vi "WebServiceLoop.vi"(8 "Error In":errorcluster, 11 "Message Queues":T1) -> (0 "Error Out":errorcluster)   [LabVIEW 2017, in "Server.lvlib" / "WebServiceCommunication.lvlib"]
doc: "This Loop sets, reads and calls the WebServiceFGV.vi which is responsible for communicating with the Webservice Methods.\nThis Loop has a timeout on the queue read function and will call the \"CheckClients\"-mode of the FGV frequently to validate which clients are still sending their heartbeat.\nIt is waiting for Messages in the WebServ-Queue and forwards messages (such as current clients connected to the MHL)."
uses:
  WebServiceCommunication.lvlib
  Message Queue/CommReferences.ctl
  Message Queue/MessageCluster.ctl
  WebServiceLoopData.ctl
  TypeDefs/ClientConfiguration.ctl
  WebServiceFGVcommands.ctl
  TypeDefs/SR List.ctl
  TypeDefs/SR Data.ctl
  TypeDefs/ServerINI.ctl
  Oracle/OracleData.ctl
  <vilib>/Utility/error.llb/Error Cluster From Error Code.vi
  Message Queue/EnqueueMessage(Single).vi
  <vilib>/ErrorRing/Error Ring.xnode
  Message Queue/Message Queue.lvlib
  Server.lvlib
  ErrorLogger/ErrorLogger.lvlib
  Oracle/Oracle.lvlib
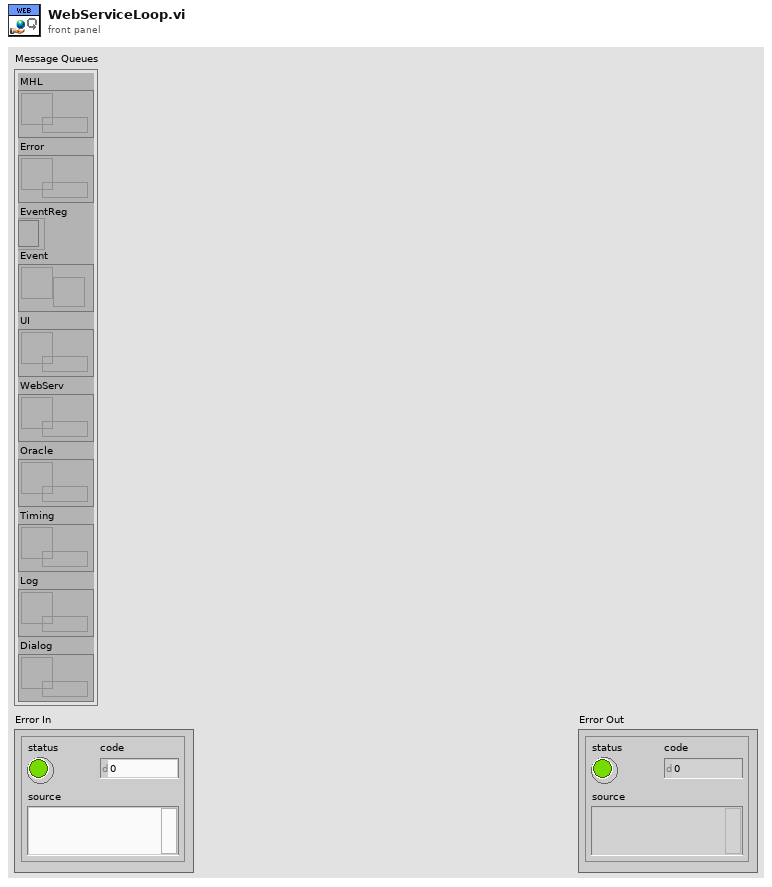
[diagram p1: front panel]
types:
  T1 = typedef "Server.lvlib/Message Queue.lvlib/CommReferences.ctl" = cluster{"MHL":refnum<queue>, "Error":refnum<queue>, "EventReg":refnum<event-registration>, "Event":refnum<user-event>, "UI":refnum<queue>, "WebServ":refnum<queue>, "Oracle":refnum<queue>, "Timing":refnum<queue>, "Log":refnum<queue>, "Dialog":refnum<queue>}
  T2 = typedef "Server.lvlib/WebServiceCommunication.lvlib/WebServiceLoopData.ctl" = cluster{"ClientTimeout":u32, "ClientConfig":T3}
  T3 = typedef "Server.lvlib/ClientConfiguration.ctl" = cluster{"ColorCodes":u32[]}
  T4 = typedef "Server.lvlib/WebServiceCommunication.lvlib/WebServiceFGVcommands.ctl" = enum16{"Init", "Reset", "Heartbeat", "GetSRs", "SetSRs", "CheckClients", "GetClients", "SetClientConfig", "GetClientConfig"}
  T5 = typedef "Server.lvlib/ServerINI.ctl" = cluster{"ClientTimeout (s)":u32, "LogPath":path, "ErrorsToIgnore":i32[], "OracleData":T6, "ClientConfig":T3}
  T6 = typedef "Server.lvlib/Oracle.lvlib/OracleData.ctl" = cluster{"DBname":string, "User":string, "Password":string}
  T7 = typedef "Server.lvlib/SR List.ctl" = T8[]
  T8 = typedef "Server.lvlib/SR Data.ctl" = cluster{"SR#":dbl, "Group":string, "Owner":string, "Problem Summary":string, "Last Updated":timestamp, "Customer First Name":string, "Customer Last Name":string, "Company":string, "Created On":timestamp, "SR Type":string, "Status":string, "Service Level":string, "Channel":string, "Days Open":dbl}
  T9 = typedef "Server.lvlib/ClientList.ctl" = T10[]
  T10 = typedef "Server.lvlib/ClientData.ctl" = cluster{"ClientID":string, "LastHeartbeat":timestamp}
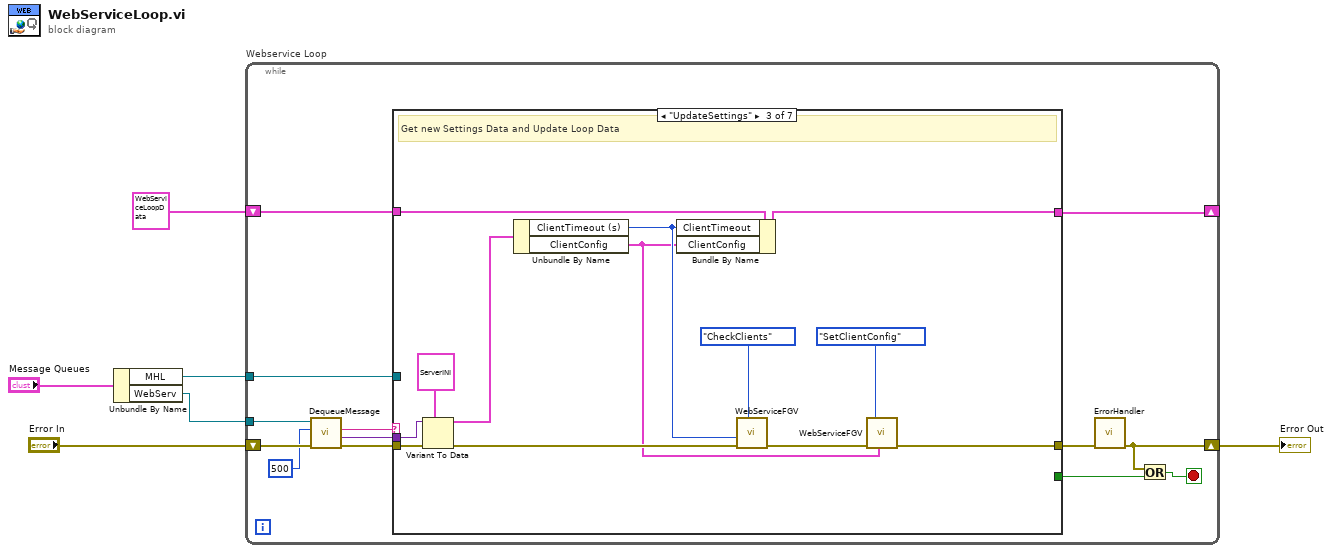
[diagram p0: block diagram]
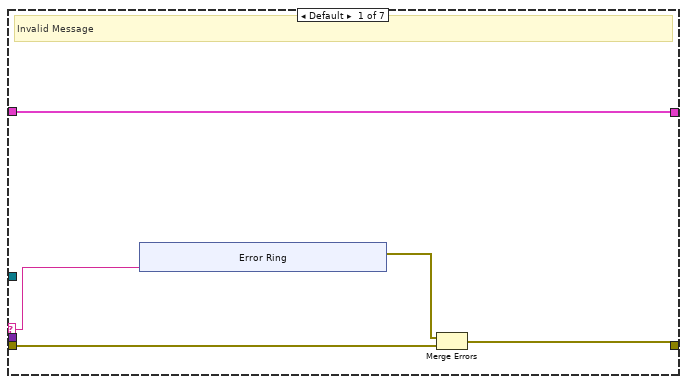
[diagram p2: hidden frame]
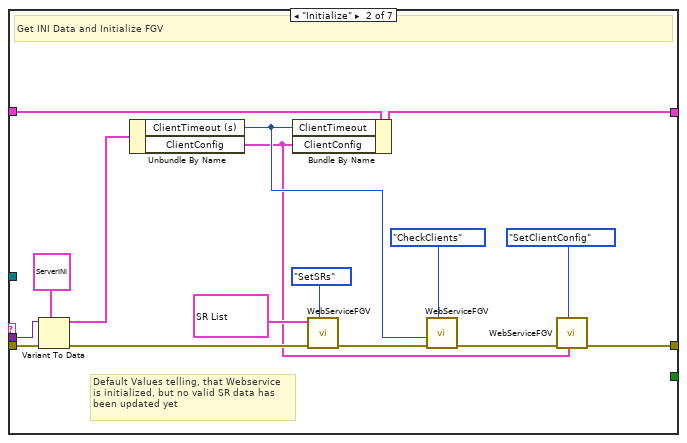
[diagram p3: hidden frame]
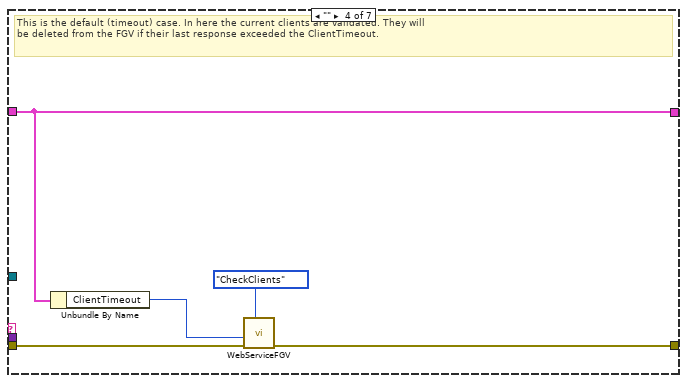
[diagram p4: hidden frame]
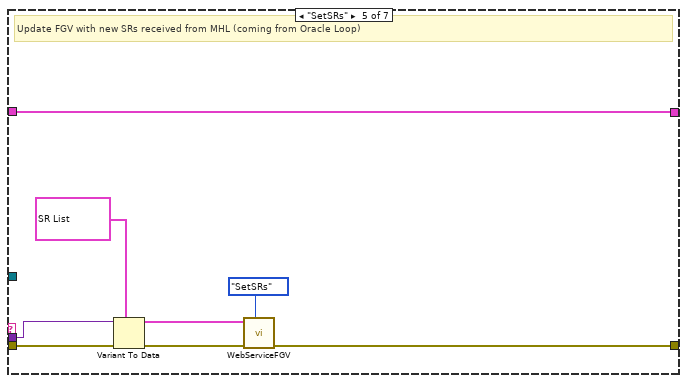
[diagram p5: hidden frame]
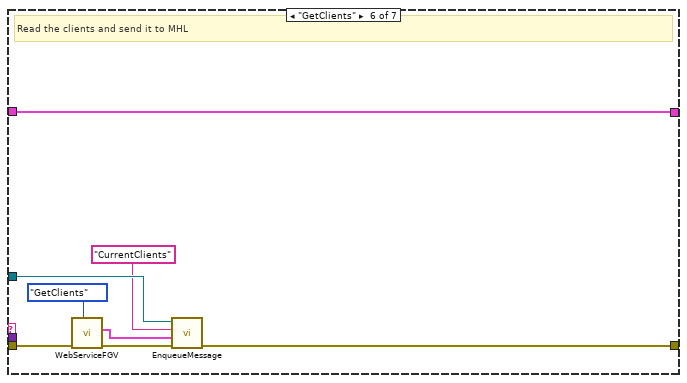
[diagram p6: hidden frame]
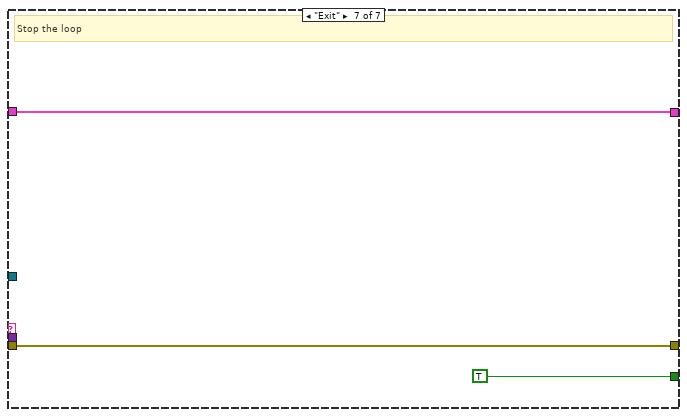
[diagram p7: hidden frame]
diagram:
  n1 = Unbundle By Name("Message Queues") -> ("MHL"=w2:refnum<queue>, "WebServ"=w3:refnum<queue>)
  n2 = while "Webservice Loop" {
    shift-right: [w7] -> w5
    shift-left: "Error In" -> [w19]
    tunnel: w3 -> [w16]
    tunnel: w2 -> [w11]
    shift-right: [w9] -> _
    shift-left: T2 {"ClientTimeout"=0, "ClientConfig"={"ColorCodes"=[16711680, 6618880, 16774745, 9567230]}} ("WebServiceLoopData") -> [w10]
    stop <- w8 stop-if-true
    n3 = call "DequeueMessage.vi"("error in (no error)"=w19, "timeout ms (-1)"=500, "Message Queue"=w16) -> ("error out"=w17:errorcluster, "Message Data"=w14:variant, "Message"=w15:string)  [unwired: 4 in, 2 out]
    n4 = case shown="\"UpdateSettings\"" w15 {
      selector: w15 -> [w21 _ _ _ _ _ _]
      tunnel: [w23 w34 w50 w61 w72 w78 w84] -> w18
      tunnel: w17 -> [w24 w47 w60 w65 w73 w81 w84]
      tunnel: w14 -> [_ w39 w57 _ w70 _ _]
      tunnel: [_ _ _ _ _ _ TRUE] -> w13
      tunnel: w11 -> [_ _ _ _ _ w77 _]
      tunnel: [w20 w38 w56 w63 w66 w74 w82] -> w9
      tunnel: w10 -> [w20 w42 w59 w63 w66 w74 w82]
      frame Default {
        # "Invalid Message"
        n5 = xnode "Error Ring"("parameter 0"=w21) -> ("error out"=w22:errorcluster)
        n6 = Merge Errors(w22, w24) -> (w23:errorcluster)
      }
      frame "Initialize" {
        # "Default Values telling, that Webservice\nis initialized, but no valid SR data has\nbeen updated yet"
        # "Get INI Data and Initialize FGV"
        n7 = Variant To Data(error in=w47, type=T5 {"ClientTimeout (s)"=30, "LogPath"=path "C:/Users/jgoebel/Documents/GitHub/AEDashboard/ServerLib/Data/ServerLog.tdms", "ErrorsToIgnore"=[], "OracleData"={"DBname"="", "User"="", "Password"=""}, "ClientConfig"={"ColorCodes"=[16711680, 6618880, 16774745, 9567230]}} ("ServerINI"), Variant=w39) -> (data=w37:T5, error out=w41:errorcluster)
        n8 = Unbundle By Name(w37) -> ("ClientTimeout (s)"=w36:u32, "ClientConfig"=w33:T3)
        n9 = Bundle By Name(cluster=w42, "ClientTimeout"=w36, "ClientConfig"=w33) -> (w38:T2)
        n10 = call "WebServiceFGV.vi"("CMD"=WebServiceFGVcommands."SetSRs", "error in (no error)"=w41, "SRListIn"=T7 [{"SR#"=1234.0, "Group"="THIS IS A DUMMY SR!", "Owner"="WEBSERVER IS INITIALIZED!", "Problem Summary"="BUT NO VALID SR DATA IS SET YET!", "Last Updated"=timestamp(0 s since 1904-01-01), "Customer First Name"="", "Customer Last Name"="", "Company"="", "Created On"=timestamp(0 s since 1904-01-01), "SR Type"="", "Status"="", "Service Level"="", "Channel"="", "Days Open"=0.0}]) -> ("error out"=w44:errorcluster)  [unwired: 5 in, 3 out]
        n11 = call "WebServiceFGV.vi"("CMD"=WebServiceFGVcommands."CheckClients", "error in (no error)"=w44, "ClientTimeout(s)(30)"=w36) -> ("error out"=w35:errorcluster)  [unwired: 5 in, 3 out]
        n12 = call "WebServiceFGV.vi"("ClientConfig"=w33, "CMD"=WebServiceFGVcommands."SetClientConfig", "error in (no error)"=w35) -> ("error out"=w34:errorcluster)  [unwired: 5 in, 3 out]
      }
      frame "UpdateSettings" {
        # "Get new Settings Data and Update Loop Data"
        n13 = Variant To Data(error in=w60, type=T5 {"ClientTimeout (s)"=30, "LogPath"=path "C:/Users/jgoebel/Documents/GitHub/AEDashboard/ServerLib/Data/ServerLog.tdms", "ErrorsToIgnore"=[], "OracleData"={"DBname"="", "User"="", "Password"=""}, "ClientConfig"={"ColorCodes"=[16711680, 6618880, 16774745, 9567230]}} ("ServerINI"), Variant=w57) -> (data=w55:T5, error out=w51:errorcluster)
        n14 = Unbundle By Name(w55) -> ("ClientTimeout (s)"=w49:u32, "ClientConfig"=w48:T3)
        n15 = Bundle By Name(cluster=w59, "ClientTimeout"=w49, "ClientConfig"=w48) -> (w56:T2)
        n16 = call "WebServiceFGV.vi"("CMD"=WebServiceFGVcommands."CheckClients", "error in (no error)"=w51, "ClientTimeout(s)(30)"=w49) -> ("error out"=w54:errorcluster)  [unwired: 5 in, 3 out]
        n17 = call "WebServiceFGV.vi"("ClientConfig"=w48, "CMD"=WebServiceFGVcommands."SetClientConfig", "error in (no error)"=w54) -> ("error out"=w50:errorcluster)  [unwired: 5 in, 3 out]
      }
      frame "" {
        # "This is the default (timeout) case. In here the current clients are validated. They will\nbe deleted from the FGV if their last response exceeded the ClientTimeout."
        n18 = Unbundle By Name(w63) -> ("ClientTimeout"=w62:u32)
        n19 = call "WebServiceFGV.vi"("CMD"=WebServiceFGVcommands."CheckClients", "error in (no error)"=w65, "ClientTimeout(s)(30)"=w62) -> ("error out"=w61:errorcluster)  [unwired: 5 in, 3 out]
      }
      frame "SetSRs" {
        # "Update FGV with new SRs received from MHL (coming from Oracle Loop)"
        n20 = Variant To Data(error in=w73, type=T7 [{"SR#"=0.0, "Group"="", "Owner"="", "Problem Summary"="", "Last Updated"=timestamp(0 s since 1904-01-01), "Customer First Name"="", "Customer Last Name"="", "Company"="", "Created On"=timestamp(0 s since 1904-01-01), "SR Type"="", "Status"="", "Service Level"="", "Channel"="", "Days Open"=0.0}] ("SRListIn"), Variant=w70) -> (data=w68:T7, error out=w71:errorcluster)
        n21 = call "WebServiceFGV.vi"("CMD"=WebServiceFGVcommands."SetSRs", "error in (no error)"=w71, "SRListIn"=w68) -> ("error out"=w72:errorcluster)  [unwired: 5 in, 3 out]
      }
      frame "GetClients" {
        # "Read the clients and send it to MHL"
        n22 = call "WebServiceFGV.vi"("CMD"=WebServiceFGVcommands."GetClients", "error in (no error)"=w81) -> ("error out"=w80:errorcluster, "ClientList"=w75:T9)  [unwired: 6 in, 2 out]
        n23 = call-poly "EnqueueMessage.vi"("error in (no error)"=w80, "Message Data"=w75, "Message"="CurrentClients", "Message Queue"=w77) -> ("error out"=w78:errorcluster)  [unwired: 6 in, 1 out]
      }
      frame "Exit" {
        # "Stop the loop"
      }
    }
    n24 = call "ErrorHandler.vi"("error in (no error)"=w18) -> ("error out"=w7:errorcluster)  [unwired: 10 in]
    n25 = Or(x=w7, y=w13) -> (x .or. y?=w8:bool)
  }
  "Error Out" <- w5
